vi "Activate-timing-source.vi"(8 "error in":errorcluster, 11 "Data ref. in":refnum<data-value>) -> (0 "error IO":errorcluster, 3 "Data ref.":refnum<data-value>, 5 "Succes?":bool)   [LabVIEW 2013, in "CameraVision.lvlib" / "CV-Main.lvclass"]
uses:
  CV-Main.lvclass
  UI/Module-states.ctl
  UI/Popup-messages.ctl
  CV-Main.lvclass/CV-Main.ctl
  Acquisition/CV-Acquisition.lvclass/CV-Acquisition.ctl
  Read Acquis params.vi
  Acquisition/Read Maximum frame rate.vi
  Acquisition/Read External timing channel.vi
  Acquisition/Read Trigger mode.vi
  Acquisition/Read Precision hardware counter.vi
  Acquisition/Read Manual trigger ID.vi
  Acquisition/Read External gating channel.vi
  Acquisition/Write Timing source.vi
  Acquisition/Write Timing source period.vi
  Acquisition/Write Gate source.vi
  <vilib>/DAQmx/create/channels.llb/DAQmx Create Channel (DI-Digital Input).vi
  <vilib>/DAQmx/create/timing.llb/DAQmx Create Timing Source (Digital Edge using Counter).vi
  <vilib>/Platform/TimedLoop/scheduler/LVUserAPI/_suppVIs/Create_SoftwareTrigger_TSource.vi
  <vilib>/Platform/TimedLoop/scheduler/LVUserAPI/_suppVIs/Create_1kHz_TSource.vi
  <vilib>/DAQmx/create/timing.llb/DAQmx Create Timing Source (Frequency).vi
  Acquisition/CV-Acquisition.lvclass
  UI/CV-UI.lvclass
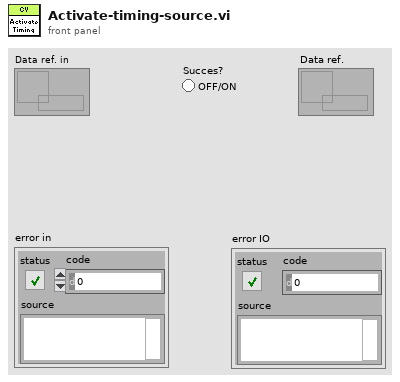
[diagram p1: front panel]
types:
  T1 = typedef "CameraVision.lvlib/CV-UI.lvclass/Popup-messages.ctl" = enum16{"Error-Black image", "Error-Camera config file", "Error-Camera connect", "Error-Grabber init", "Error-Camera setting", "Error-Image offset", "Error-Image import", "Error-Settings file not exist", "Error-Timing source", "Conflict-Filters", "Conflict-Map", "Conflict-Framerate", "Conflict-Charact", "Conflict-Temperature field", "Conflict-Temperature value", "Conflict-Storage-Binary image", "Conflict-Storage-Corrected image", "Conflict-Storage-Map", "Conflict-Storage-Charact", "Conflict-Storage-Temperature field", "Conflict-Storage-Temperature value", "Warning-File exist", "Warning-Parameter reset", "Warning-User cancel", "Info-Images imported"}
  T2 = typedef "CameraVision.lvlib/CV-UI.lvclass/Module-states.ctl" = enum16{"Inactive", "Active", "Data-loss", "Error", "Simulation", "Synchronizing", "Initialized", "Released"}
  T3 = typedef "Trigger-modes.ctl" = enum16{"Camera timed (not sync.)", "Framegrabber timed (sync.)", "Software timed (sync.)", "External timing (sync.)", "Manual (sync.)", "Gated - camera (not sync.)", "Gated - grabber (sync.)", "Gated - software (sync.)", "Gated - external (sync.)"}
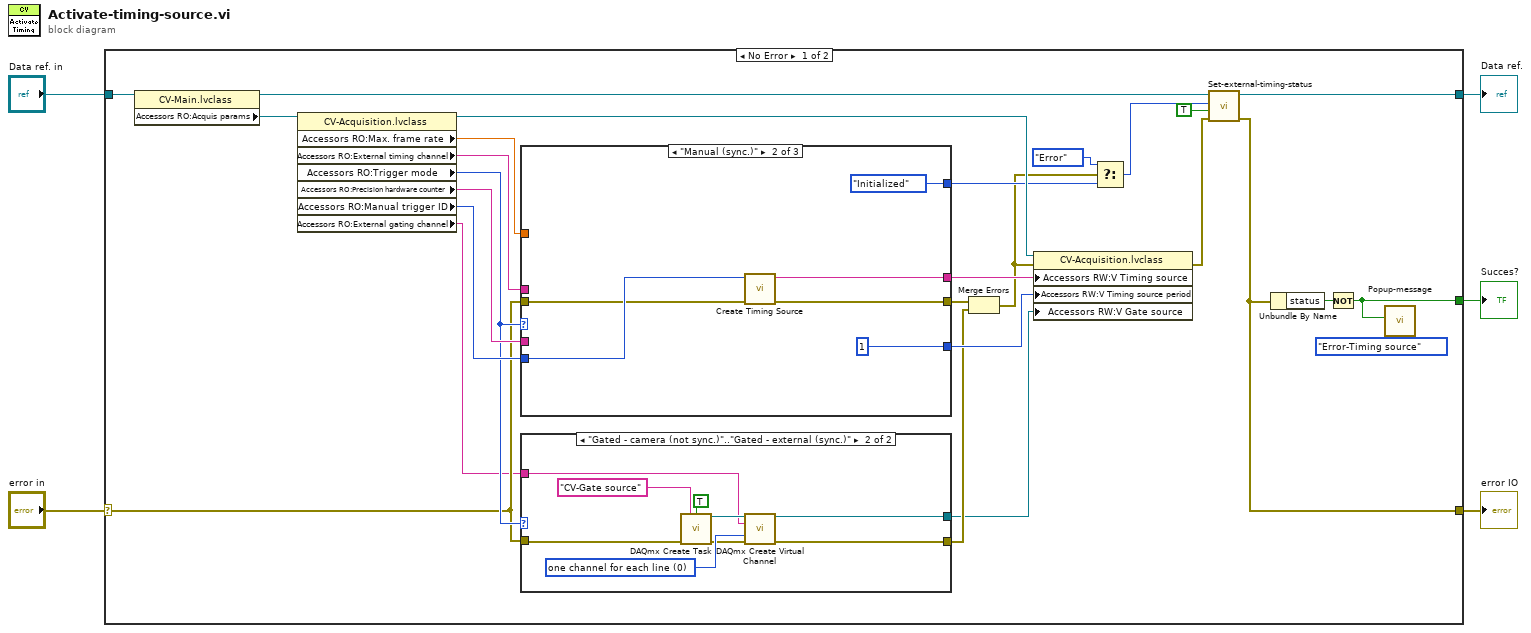
[diagram p0: block diagram]
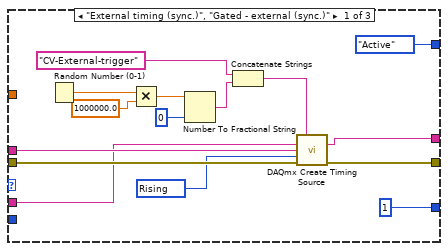
[diagram p3: hidden frame]
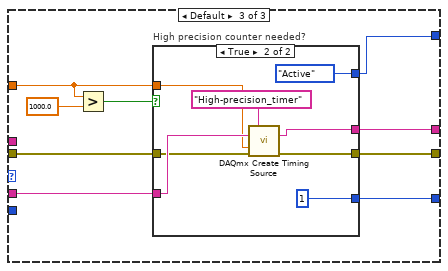
[diagram p4: hidden frame]
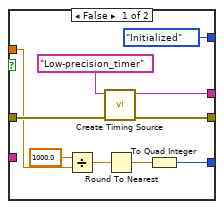
[diagram p5: hidden frame]
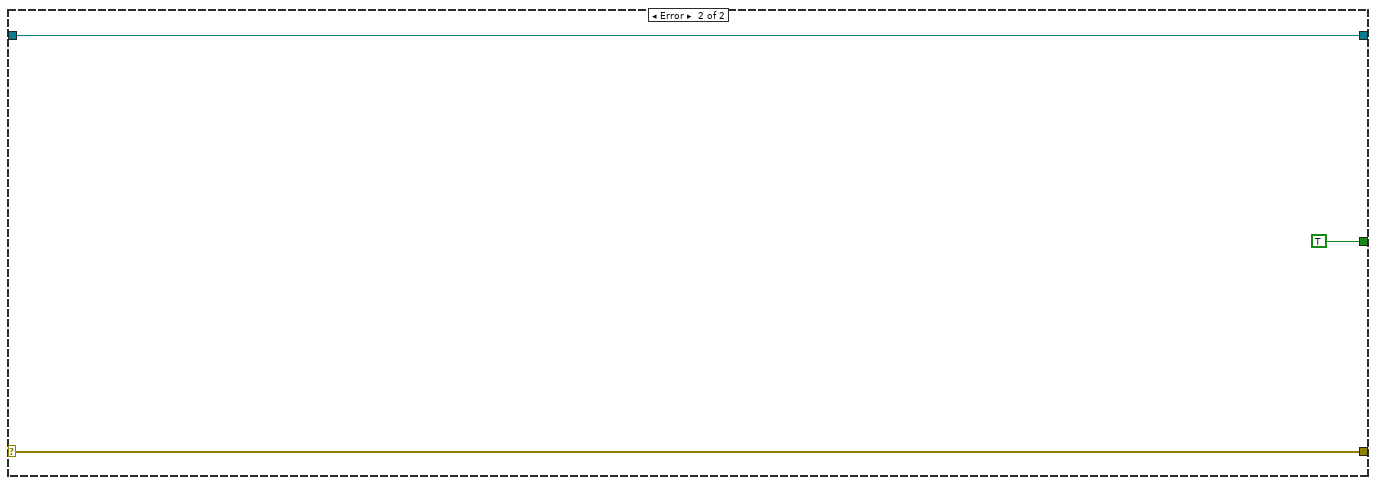
[diagram p6: hidden frame]
diagram:
  n1 = case shown="No Error" "error in" {
    selector: "error in" -> [w18 w93]
    tunnel: "Data ref. in" -> [w15 w92]
    tunnel: [w6 w93] -> w3
    tunnel: [w10 w92] -> w2
    tunnel: [w16 TRUE] -> w1
    frame No Error {
      n2 = property class="CV-Main.lvclass"(reference=w15) -> (reference out=w11:refnum<data-value>, "Accessors RO:Acquis params"=w23:refnum<data-value>)  [unwired: 1 in, 1 out]
      n3 = property class="CV-Acquisition.lvclass"(reference=w23) -> (reference out=w30:refnum<data-value>, "Accessors RO:Max. frame rate"=w26:dbl, "Accessors RO:External timing channel"=w9:tag, "Accessors RO:Trigger mode"=w19:T3, "Accessors RO:Precision hardware counter"=w32:tag, "Accessors RO:Manual trigger ID"=w31:u8, "Accessors RO:External gating channel"=w17:tag)  [unwired: 1 in, 1 out]
      n4 = case shown="\"Manual (sync.)\"" w19 {
        tunnel: w26 -> [_ _ w68]
        tunnel: w32 -> [w51 _ w70]
        tunnel: w18 -> [w55 w60 w69]
        tunnel: [w57 w62 w67] -> w29
        tunnel: [w56 w63 w66] -> w22
        tunnel: w9 -> [w52 _ _]
        tunnel: w31 -> [_ w61 _]
        tunnel: [i64 1 i64 1 w65] -> w27
        tunnel: [Module-states."Active" ("Timing status") Module-states."Initialized" ("Timing status") w64] -> w24
        frame "External timing (sync.)", "Gated - external (sync.)" {
          w50 = 10280 items=["Rising"=10280, "Falling"=10171] ("edge")
          n5 = Random Number (0-1)() -> (number: 0 to 1=w49:dbl)
          n6 = Multiply(x=w49, y=1000000.0) -> (x*y=w47:dbl)
          n7 = Number To Fractional String(number=w47, precision (6)=i16 0) -> (F-format string=w45:string)  [unwired: 2 in]
          n8 = Concatenate Strings("CV-External-trigger" ("timing source name"), w45) -> (w43:string)
          n9 = call-poly <vilib>:"DAQmx Create Timing Source.vi"("timing source name"=w43, "counter"=w51, "source"=w52, "edge"=w50, "error in"=w55) -> ("timing source out"=w57:string, "error out"=w56:errorcluster)  [unwired: 9 in]
        }
        frame "Manual (sync.)" {
          n10 = call-poly <vilib>:"Create Timing Source.vi"("error in (no error)"=w60, "trigger ID"=w61) -> ("error out"=w63:errorcluster, "timing source name"=w62:string)  [unwired: 8 in]
        }
        frame Default {
          n11 = Greater?(x=w68, y=1000.0) -> (0:w71:bool)
          n12 = case "High precision counter needed?" shown="True" w71 {
            tunnel: w70 -> [_ w89]
            tunnel: [w82 w86] -> w67
            tunnel: [w81 w90] -> w66
            tunnel: w69 -> [w80 w87]
            tunnel: w68 -> [w79 w88]
            tunnel: [w76 i64 1] -> w65
            tunnel: [Module-states."Initialized" ("Timing status") Module-states."Active" ("Timing status")] -> w64
            frame False {
              n13 = Divide(x=1000.0, y=w79) -> (x/y=w77:dbl)
              n14 = call-poly <vilib>:"Create Timing Source.vi"("error in (no error)"=w80, "name (in)"="Low-precision_timer") -> ("error out"=w81:errorcluster, "name (out)"=w82:string)  [unwired: 8 in]
              n15 = Round To Nearest(number=w77) -> (nearest integer value=w73:dbl)
              n16 = To Quad Integer(1:w73) -> (0:w76:i64)
            }
            frame True {
              n17 = call-poly <vilib>:"DAQmx Create Timing Source.vi"("timing source name"="High-precision_timer", "counter"=w89, "frequency"=w88, "error in"=w87) -> ("timing source out"=w86:string, "error out"=w90:errorcluster)  [unwired: 10 in]
            }
          }
        }
      }
      n18 = case shown="\"Gated - camera (not sync.)\"..\"Gated - external (sync.)\"" w19 {
        tunnel: [w33 w37] -> w21
        tunnel: [_ w36] -> w20
        tunnel: w18 -> [w33 w35]
        tunnel: w17 -> [_ w34]
        frame Default {
        }
        frame "Gated - camera (not sync.)".."Gated - external (sync.)" {
          w42 = 0 items=["one channel for each line", "one channel for all lines"] ("line grouping")
          n19 = call <vilib>:"DAQmx Create Task.vi"("new task name"="CV-Gate source", "auto cleanup"=TRUE, "error in"=w35) -> ("task out"=w38:refnum<k21>, "error out"=w41:errorcluster)  [unwired: 11 in]
          n20 = call-poly <vilib>:"DAQmx Create Virtual Channel.vi"("task in"=w38, "lines"=w34, "line grouping"=w42, "error in"=w41) -> ("task out"=w36:refnum<k21>, "error out"=w37:errorcluster)  [unwired: 10 in]
        }
      }
      n21 = Merge Errors(w22, w21) -> (w14:errorcluster)
      n22 = property class="CV-Acquisition.lvclass"(reference=w30, error in=w14, "Accessors RW:V Timing source"=w29, "Accessors RW:V Timing source period"=w27, "Accessors RW:V Gate source"=w20) -> (error out=w13:errorcluster)  [unwired: 1 out]
      n23 = Select(t=Module-states."Error" ("Timing status"), s=w14, f=w24) -> (s? t:f=w12:T2)
      n24 = call "Set-external-timing-status.vi"("error in"=w13, "Reset errors?"=TRUE, "Timing status in"=w12, "Data ref. in"=w11) -> ("error IO"=w6:errorcluster, "Data ref."=w10:refnum<data-value>)  [unwired: 5 in, 1 out]
      n25 = Unbundle By Name(w6) -> ("status"=w28:bool)
      n26 = Not(x=w28) -> (.not. x?=w16:bool)
      n27 = call "Popup-message.vi"("Message"=Popup-messages."Error-Timing source", "Ignore?"=w16) -> ()  [unwired: 9 in, 1 out]
    }
    frame Error {
    }
  }
  "error IO" <- w3
  "Data ref." <- w2
  "Succes?" <- w1
